vi "Status Lights Spikes.vi"(1 "Light  2":bool, 2 "Light 1":bool, 3 "Mode":enum8{"Start", "Run", "Finish"}(ring)) -> ()   [LabVIEW 2014]
uses:
  <vilib>/Rock Robotics/SystemInterfaces/DIO/FPGA_DIORelayChannel.ctl
  <vilib>/Rock Robotics/WPI/Relay/WPI_RelayDirection.ctl
  <vilib>/Rock Robotics/WPI/Relay/WPI_RelayValue.ctl
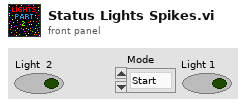
[diagram p1: front panel]
types:
  T1 = typedef "FPGA_DIORelayChannel.ctl" = enum8{"Relay 0", "Relay 1", "Relay 2", "Relay 3", "Invalid"}
  T2 = typedef "WPI_RelayDirection.ctl" = enum16{"Both directions", "Forward only", "Reverse only"}
  T3 = typedef "WPI_RelayValue.ctl" = enum16{"Off", "On", "Forward", "Reverse"}
  T4 = typedef "WPI_RelayDevRef.ctl" = cluster{"DevStatus":errorcluster, "Relay Channel":T1, "Controller":T5, "Relay Direction":T2}
  T5 = typedef "FPGA_TypedefDigitalModule.ctl" = enum16{"Controller 1"}
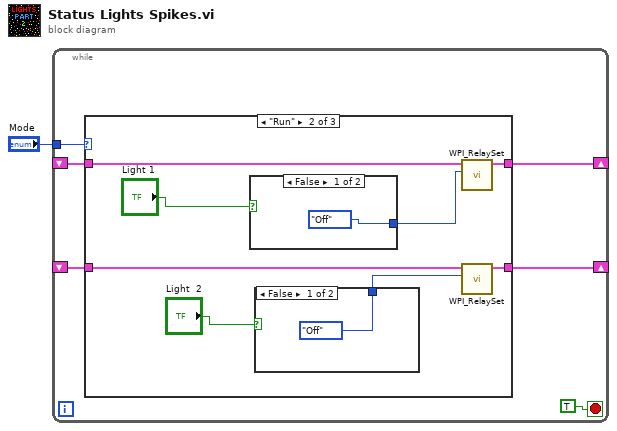
[diagram p0: block diagram]
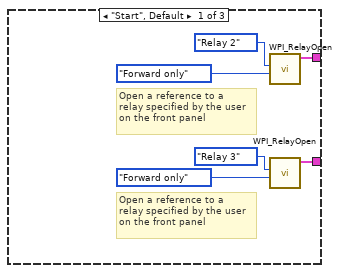
[diagram p2: hidden frame]
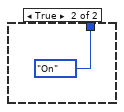
[diagram p3: hidden frame]
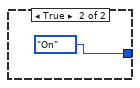
[diagram p4: hidden frame]
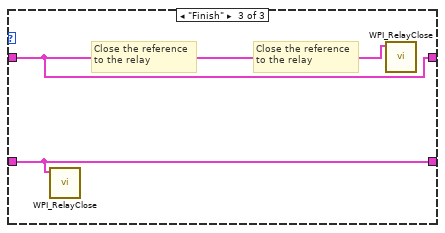
[diagram p5: hidden frame]
diagram:
  n1 = while {
    tunnel: "Mode" -> [w6]
    shift-right: [w5] -> _
    shift-left: _ -> [w4]
    shift-right: [w3] -> _
    shift-left: _ -> [w2]
    stop <- TRUE stop-if-true
    n2 = case shown="\"Run\"" w6 {
      tunnel: [w11 w20 w27] -> w5
      tunnel: w4 -> [_ w21 w27]
      tunnel: [w8 w18 w26] -> w3
      tunnel: w2 -> [_ w19 w26]
      frame "Start", Default {
        # "Open a reference to a \nrelay specified by the user\non the front panel"
        # "Open a reference to a \nrelay specified by the user\non the front panel"
        n3 = call <vilib>:"WPI_RelayOpen.vi"("Relay Direction"=WPI_RelayDirection."Forward only" ("RelayDirection"), "Relay Channel"=FPGA_DIORelayChannel."Relay 2" ("RelayChannel")) -> ("RelayDevRef"=w11:T4)  [unwired: 2 in, 7 out]
        n4 = call <vilib>:"WPI_RelayOpen.vi"("Relay Direction"=WPI_RelayDirection."Forward only" ("RelayDirection"), "Relay Channel"=FPGA_DIORelayChannel."Relay 3" ("RelayChannel")) -> ("RelayDevRef"=w8:T4)  [unwired: 2 in, 7 out]
      }
      frame "Run" {
        n5 = case shown="False" "Light 1" {
          tunnel: [WPI_RelayValue."Off" ("RelayValue") WPI_RelayValue."On" ("RelayValue")] -> w14
          frame False {
          }
          frame True {
          }
        }
        n6 = case shown="False" "Light  2" {
          tunnel: [WPI_RelayValue."Off" ("RelayValue") WPI_RelayValue."On" ("RelayValue")] -> w15
          frame False {
          }
          frame True {
          }
        }
        n7 = call <vilib>:"WPI_RelaySet.vi"("RelayValue"=w14, "RelayDevRef"=w21) -> ("RelayDevRef"=w20:T4)  [unwired: 1 in, 8 out]
        n8 = call <vilib>:"WPI_RelaySet.vi"("RelayValue"=w15, "RelayDevRef"=w19) -> ("RelayDevRef"=w18:T4)  [unwired: 1 in, 8 out]
      }
      frame "Finish" {
        # "Close the reference\nto the relay"
        # "Close the reference\nto the relay"
        n9 = call <vilib>:"WPI_RelayClose.vi"("RelayDevRef"=w26) -> ()  [unwired: 1 in, 10 out]
        n10 = call <vilib>:"WPI_RelayClose.vi"("RelayDevRef"=w27) -> ()  [unwired: 1 in, 10 out]
      }
    }
  }
